vi "Key down test.vi"() -> ()   [LabVIEW 2013]
uses:
  <vilib>/event_ctls.llb/eventvkey.ctl
  <vilib>/Utility/inputDevices.llb/keyboardAcquire.vi
  <vilib>/Utility/inputDevices.llb/closeKeyboard.vi
panel:
  out "Char":i16
  out "Boolean":bool
  out "keys pressed":T1(array[ring])
  in  "stop":bool
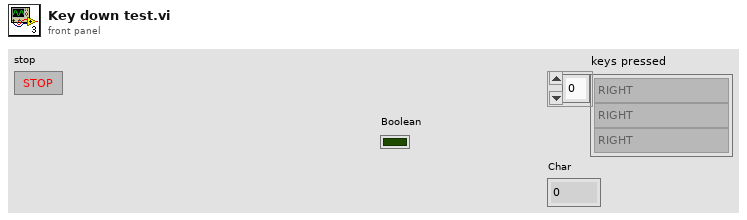
[diagram p1: front panel]
types:
  T1 = enum16{"0", "1", "2", "3", "4", "5", "6", "7", "8", "9", "A", "B", "C", "D", "E", "F", "G", "H", "I", "J", "K", "L", "M", "N", "O", "P", "Q", "R", "S", "T", "U", "V", "W", "X", "Y", "Z", "F1", "F2", "F3", "F4", "F5", "F6", "F7", "F8", "F9", "F10", "F11", "F12", "F13", "F14", "F15", "ADD", "BACK", "BACKSLASH", "CAPITAL", "COMMA", "DECIMAL", "DELETE", "DIVIDE", "DOWN", "END", "EQUALS", "ESCAPE", "GRAVE (`)", "HOME", "INSERT", "LBRACKET", "LCONTROL", "LEFT", "L ALT", "LSHIFT", "LWIN", "MINUS", "MULTIPLY", "NEXT", "NUMLOCK", "NUMPAD_0", "NUMPAD_1", "NUMPAD_2", "NUMPAD_3", "NUMPAD_4", "NUMPAD_5", "NUMPAD_6", "NUMPAD_7", "NUMPAD_8", "NUMPAD_9", "PAUSE", "PERIOD", "PRIOR (PG UP)", "RBRACKET", "RCONTROL", "RETURN", "RIGHT", "R ALT", "RSHIFT", "RWIN", "SCROLL", "SEMICOLON", "SLASH", "SPACE", "SUBTRACT", "TAB", "UP", "ENTER (num pad)", "' (quote)"}[]
  T2 = typedef "eventvkey.ctl" = enum16{"ASCII", "Enter", "Return", "Shift", "Ctrl", "Alt", "Cmd", "Opt", "Caps", "NumLock", "Clear", "Break", "Up", "Down", "Left", "Right", "Insert", "Delete", "Home", "End", "PageUp", "PageDown", "Escape", "Help", "Pause", "ScrollLock", "F1", "F2", "F3", "F4", "F5", "F6", "F7", "F8", "F9", "F10", "F11", "F12", "F13", "F14", "F15", "F16", "F17", "F18", "F19", "F20", "F21", "F22", "F23", "F24", "Play", "VolumeUp", "VolumeDown", "Mute", "Two Byte Char"}
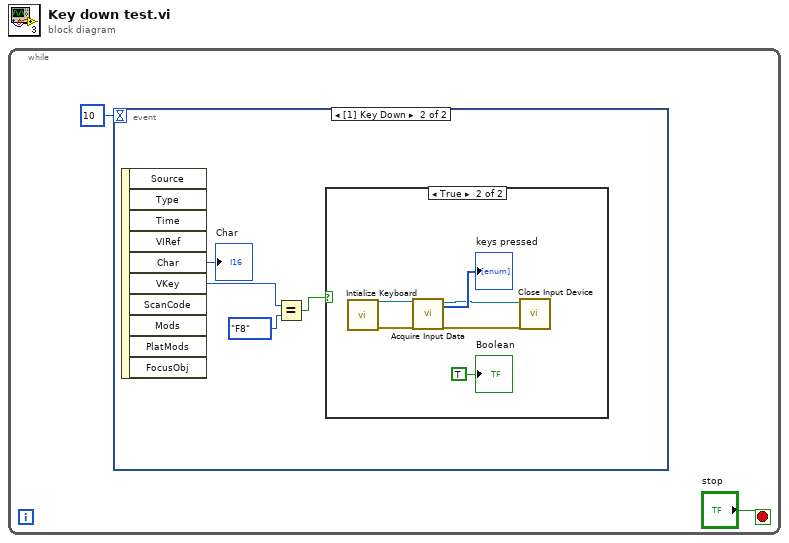
[diagram p0: block diagram]
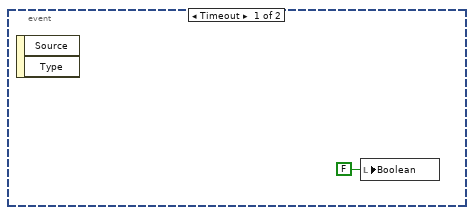
[diagram p2: hidden frame]
diagram:
  n1 = while {
    stop <- "stop" stop-if-true
    n2 = event shown="[1] Key Down" {
      selector: _ -> [_ _]
      dyn-events: _ -> [_ _]
      timeout: 10 -> [_ _]
      event Timeout {
        n3 = event-data() -> ()  [unwired: 1 in, 2 out]
        n4 = local write "Boolean"(FALSE ("Boolean")) -> ()
      }
      event Key Down {
        n5 = event-data() -> ("Char"=→"Char":i16, "VKey"=w7:T2)  [unwired: 1 in, 8 out]
        n6 = Equal?(x=w7, y=eventvkey."F8" ("VKey")) -> (x = y?=w5:bool)
        n7 = case shown="True" w5 {
          frame False {
          }
          frame True {
            n8 = call <vilib>:"Intialize Keyboard.vi"() -> ("error out"=w12:errorcluster, "device ID"=w13:refnum<k1>)  [unwired: 10 in]
            n9 = call-poly <vilib>:"Acquire Input Data.vi"("device ID"=w13, "error in (no error)"=w12) -> ("device ID"=w10:refnum<k1>, "keys pressed"=→"keys pressed":T1, "error out"=w9:errorcluster)  [unwired: 15 in]
            n10 = call-poly <vilib>:"Close Input Device.vi"("error in (no error)"=w9, "device ID"=w10) -> ()  [unwired: 8 in, 1 out]
            "Boolean" <- TRUE ("Boolean")
          }
        }
      }
    }
  }
